vi "PDash New Event.vi"(8 "error in":errorcluster, 10 "Current Selection":T4, 11 "Project":refnum<class "Project.lvclass">) -> (0 "error out":errorcluster)   [LabVIEW 2020]
doc: "Panther Dashboard DQMH UI Template"
uses:
  Panther Dashboard.lvlib
  Class/Library/Library.lvclass
  Class/Project/Project.lvclass
  <vilib>/Delacor/Delacor QMH/Libraries/_Scripting Support/Request Scoping--enum.ctl
  <vilib>/Delacor/Delacor QMH/Libraries/_Scripting Support/dqmh_lib_DQMH Scripting Support.lvlib
  <vilib>/Delacor/Delacor QMH/Libraries/_Scripting Support/Module Type--enum.ctl
  Controls/Cancel.ctl
  Controls/Continue.ctl
  Class/VI/VI.lvclass
  <vilib>/Delacor/Delacor QMH/Libraries/_Scripting Support/Module Info--cluster.ctl
panel:
  out "error out 2":errorcluster
  in  "Module Info":T1
  in  "Event Info":T3
  in  "error in 2":errorcluster
  in  "Pre Set Dummy Arg":bool
  in  "Progress Title (\"New DQMH Event\")":string
  in  "Skip Post-Scripting Action (F)":bool
  out "Selected Module":string caption="Current Module Selection:"
  in  "Module Description":string caption="New Module Description"
  in  "New Module Path":path
  in  "Module Name":string caption="New Module Name"
  in  "Continue":T5
  in  "Cancel":T6
  # "Note: To Select the DQMH Default UIs, click the Gear Icon on the Panther Dashboard\nMain UI, and Uncheck the 'Use Panther Dashboard UIs' checkbox."
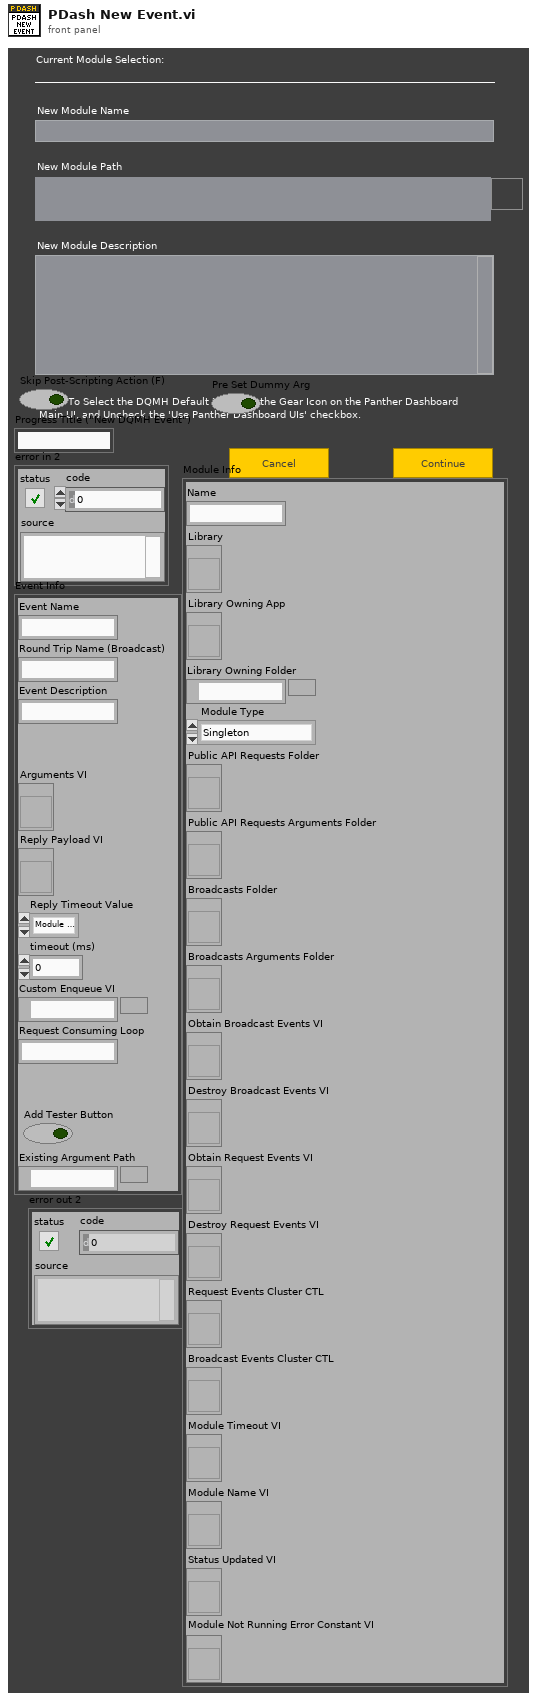
[diagram p1: front panel]
types:
  T1 = typedef "dqmh_lib_DQMH Scripting Support.lvlib/Module Info--cluster.ctl" = cluster{"Name":string, "Library":refnum<vi>, "Library Owning App":refnum<vi>, "Library Owning Folder":path, "Module Type":T2, "Public API Requests Folder":refnum<vi>, "Public API Requests Arguments Folder":refnum<vi>, "Broadcasts Folder":refnum<vi>, "Broadcasts Arguments Folder":refnum<vi>, "Obtain Broadcast Events VI":refnum<vi>, "Destroy Broadcast Events VI":refnum<vi>, "Obtain Request Events VI":refnum<vi>, "Destroy Request Events VI":refnum<vi>, "Request Events Cluster CTL":refnum<vi>, "Broadcast Events Cluster CTL":refnum<vi>, "Module Timeout VI":refnum<vi>, "Module Name VI":refnum<vi>, "Status Updated VI":refnum<vi>, "Module Not Running Error Constant VI":refnum<vi>}
  T2 = typedef "dqmh_lib_DQMH Scripting Support.lvlib/Module Type--enum.ctl" = enum16{"Singleton", "Cloneable"}
  T3 = typedef "dqmh_lib_DQMH Scripting Support.lvlib/Event Info (New)--cluster.ctl" = cluster{"Event Name":string, "Round Trip Name (Broadcast)":string, "Event Description":string, "Arguments VI":refnum<vi>, "Reply Payload VI":refnum<vi>, "Reply Timeout Value":enum32{"Module Timeout", "Custom"}, "timeout (ms)":i32, "Custom Enqueue VI":path, "Request Consuming Loop":string, "Add Tester Button":bool, "Existing Argument Path":path}
  T4 = cluster{"Library":refnum<class "Library.lvclass">, "VI":refnum<class "VI.lvclass">}
  T5 = typedef "Continue.ctl" = bool
  T6 = typedef "Cancel.ctl" = bool
  T7 = cluster{"Name":string, "Library":refnum<vi>, "Library Owning App":refnum<vi>, "Library Owning Folder":path, "Public API Requests Folder":refnum<vi>, "Public API Requests Arguments Folder":refnum<vi>, "Broadcasts Folder":refnum<vi>, "Broadcasts Arguments Folder":refnum<vi>, "Obtain Broadcast Events VI":refnum<vi>, "Destroy Broadcast Events VI":refnum<vi>, "Obtain Request Events VI":refnum<vi>, "Destroy Request Events VI":refnum<vi>, "Request Events Cluster CTL":refnum<vi>, "Broadcast Events Cluster CTL":refnum<vi>, "Module Timeout VI":refnum<vi>, "Module Name VI":refnum<vi>, "Status Updated VI":refnum<vi>, "Module Not Running Error Constant VI":refnum<vi>}
  T8 = cluster{"Event Name":string, "Round Trip Name (Broadcast)":string, "Event Description":string, "Arguments VI":refnum<vi>, "Reply Payload VI":refnum<vi>, "Reply Timeout Value":enum32{"Module Timeout", "Custom"}, "timeout (ms)":i32, "Custom Enqueue VI":path, "Request Consuming Loop":string, "Add Tester Button":bool, "Existing Argument Path":path}
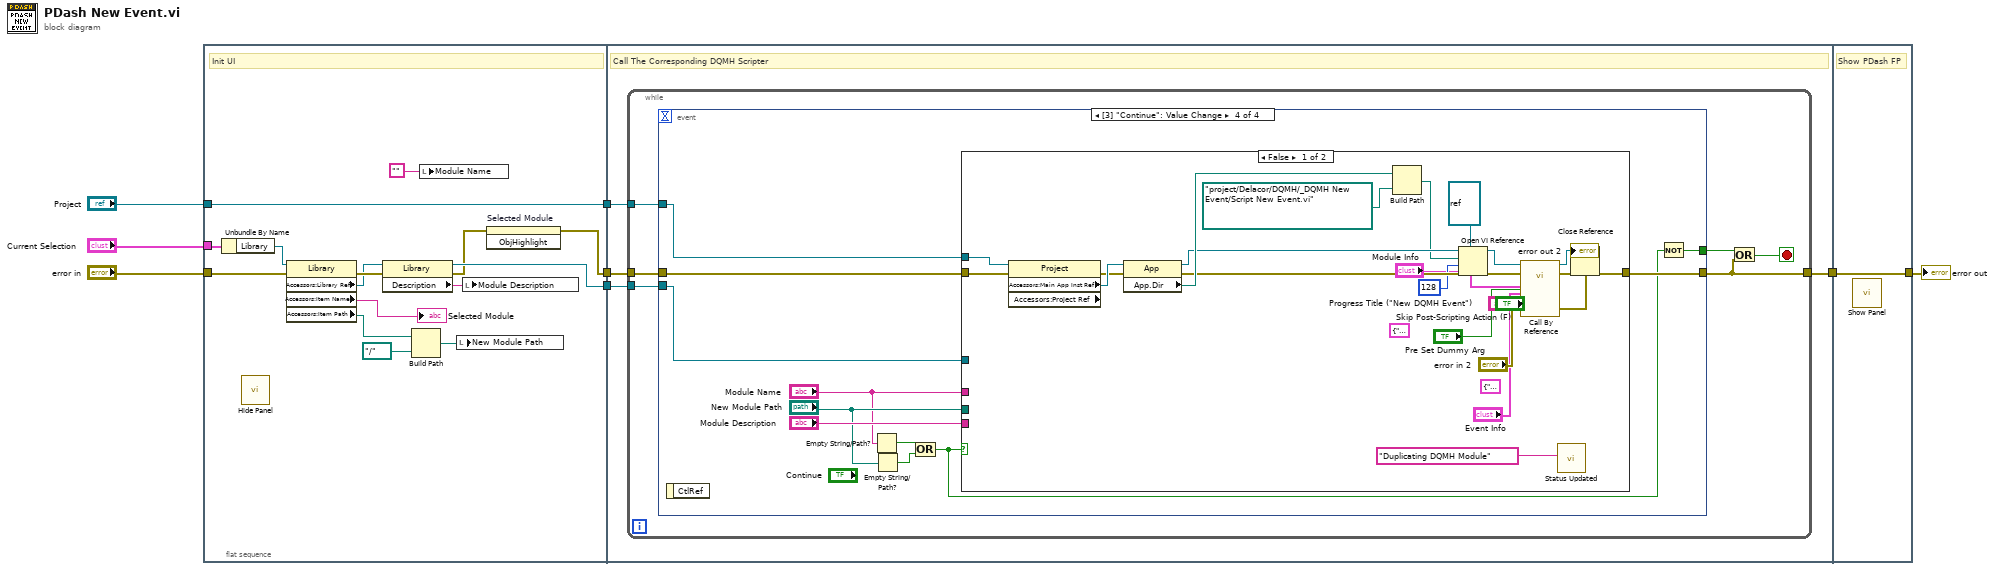
[diagram p0: block diagram]
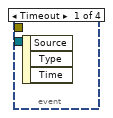
[diagram p2: hidden frame]
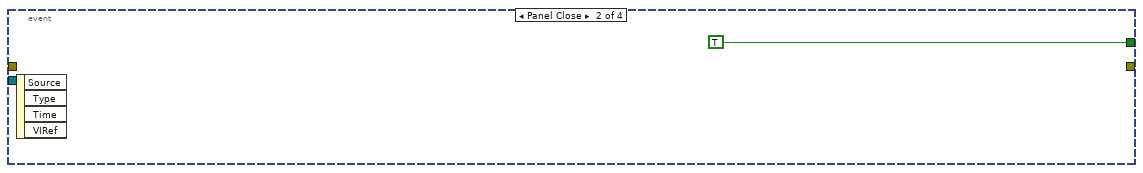
[diagram p3: hidden frame]
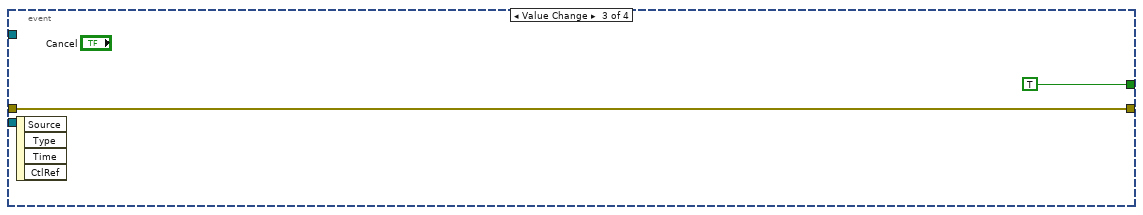
[diagram p4: hidden frame]
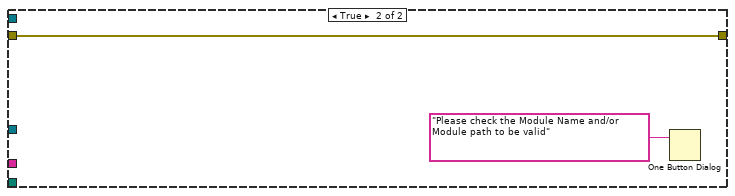
[diagram p5: hidden frame]
diagram:
  n1 = flat-sequence {
    tunnel: "Project" -> [w21]
    tunnel: [w21] -> w3
    tunnel: "error in" -> [w23]
    tunnel: [w9] -> w5
    tunnel: "Current Selection" -> [w20]
    tunnel: [w13] -> w1
    tunnel: [w27] -> w8
    tunnel: w3 -> [w25]
    tunnel: w5 -> [w26]
    tunnel: w1 -> [w24]
    tunnel: [w74] -> w7
    tunnel: w8 -> [w74]
    frame #0 {
      # "Init UI"
      n2 = Unbundle By Name(w20) -> ("Library"=w19:refnum<class "Library.lvclass">)
      n3 = call "Hide Panel.vi"() -> ()  [unwired: 11 in, 1 out]
      n4 = property class="Library"(reference=w19, error in=w23) -> (error out=w22:errorcluster, "Accessors:Library Ref"=w14:refnum<vi>, "Accessors:Item Name"=→"Selected Module":string, "Accessors:Item Path"=w16:path)  [unwired: 1 out]
      n5 = property class="Library"(reference=w14, error in=w22) -> (reference out=w13:refnum<vi>, error out=w10:errorcluster, "Description"=w12:string)
      n6 = Build Path(base path=w16, name or relative path=path "../..") -> (appended path=w18:path)
      n7 = local write "Module Name"("") -> ()
      n8 = local write "New Module Path"(w18) -> ()
      n9 = local write "Module Description"(w12) -> ()
      n10 = invoke on="Selected Module" class="Str" method="ObjHighlight"(error in=w10) -> (error out=w9:errorcluster)  [unwired: 2 in, 2 out]
    }
    frame #1 {
      # "Call The Corresponding DQMH Scripter"
      n11 = while {
        tunnel: [w28] -> w27
        tunnel: w25 -> [w31]
        tunnel: w26 -> [w33]
        tunnel: w24 -> [w30]
        stop <- w29 stop-if-true
        n12 = event shown="[3] \"Continue\": Value Change" {
          selector: _ -> [_ _ _ _]
          dyn-events: _ -> [_ _ _ _]
          timeout: _ -> [_ _ _ _]
          tunnel: [_ TRUE TRUE w45] -> w32
          tunnel: [_ _ w35 w38] -> w28
          tunnel: w31 -> [_ _ _ w41]
          tunnel: w33 -> [_ _ w35 w40]
          tunnel: w30 -> [_ _ _ w39]
          event Timeout {
            n13 = event-data() -> ()  [unwired: 1 in, 3 out]
          }
          event Panel Close {
            n14 = event-data() -> ()  [unwired: 1 in, 4 out]
          }
          event Value Change {
            n15 = event-data() -> ()  [unwired: 1 in, 4 out]
          }
          event Value Change {
            n16 = event-data() -> ()  [unwired: 1 in, 1 out]
            n17 = Empty String/Path?(string/path="Module Name") -> (empty?=w47:bool)
            n18 = Empty String/Path?(string/path="New Module Path") -> (empty?=w46:bool)
            n19 = Or(x=w47, y=w46) -> (x .or. y?=w37:bool)
            n20 = case shown="False" w37 {
              tunnel: "Module Description" -> [_ _]
              tunnel: "New Module Path" -> [_ _]
              tunnel: "Module Name" -> [_ _]
              tunnel: w41 -> [w60 _]
              tunnel: w40 -> [w59 w72]
              tunnel: w39 -> [_ _]
              tunnel: [w55 w72] -> w38
              frame False {
                (unwired) T7 {"Name"="", "Library"=refnum, "Library Owning App"=refnum, "Library Owning Folder"=path "", "Public API Requests Folder"=refnum, "Public API Requests Arguments Folder"=refnum, "Broadcasts Folder"=refnum, "Broadcasts Arguments Folder"=refnum, "Obtain Broadcast Events VI"=refnum, "Destroy Broadcast Events VI"=refnum, "Obtain Request Events VI"=refnum, "Destroy Request Events VI"=refnum, "Request Events Cluster CTL"=refnum, "Broadcast Events Cluster CTL"=refnum, "Module Timeout VI"=refnum, "Module Name VI"=refnum, "Status Updated VI"=refnum, "Module Not Running Error Constant VI"=refnum} ("Module Info")
                (unwired) T8 {"Event Name"="", "Round Trip Name (Broadcast)"="", "Event Description"="", "Arguments VI"=refnum, "Reply Payload VI"=refnum, "Reply Timeout Value"=enum."Module Timeout", "timeout (ms)"=0, "Custom Enqueue VI"=path "", "Request Consuming Loop"="", "Add Tester Button"=FALSE, "Existing Argument Path"=path ""} ("Event Info")
                n21 = property class="Project" props=["Accessors:Main App Inst Ref", "Accessors:Project Ref"](reference=w60, error in=w59) -> (error out=w64:errorcluster, "Accessors:Main App Inst Ref"=w69:refnum<vi>)  [unwired: 2 out]
                n22 = property class="App"(reference=w69, error in=w64) -> (reference out=w67:refnum<vi>, error out=w63:errorcluster, "App.Dir"=w68:path)
                n23 = Build Path(base path=w68, name or relative path=path "project/Delacor/DQMH/_DQMH New Event/Script New Event.vi") -> (appended path=w65:path)
                n24 = Open VI Reference(type specifier VI Refnum (for type only)=refnum<vi> refnum, application reference (local)=w67, vi path=w65, options=128, error in (no error)=w63) -> (vi reference=w70:refnum<vi>, error out=w61:errorcluster)  [unwired: 1 in]
                n25 = call-by-ref "?"(reference=w70, error in=w61, "Skip Post-Scripting Action (F)"="Skip Post-Scripting Action (F)", "Progress Title (\"New DQMH Event\")"="Progress Title (\"New DQMH Event\")", "Pre Set Dummy Arg"="Pre Set Dummy Arg", "error in"="error in 2", "Event Info"="Event Info", "Module Info"="Module Info") -> (reference out=w66:refnum<vi>, error out=w62:errorcluster, 0:"error out"=→"error out 2":errorcluster)  [unwired: 5 in]
                n26 = call "Status Updated.vi"("Status"="Duplicating DQMH Module") -> ()  [unwired: 10 in, 1 out]
                n27 = Close Reference(reference=w66, error in (no error)=w62) -> (error out=w55:errorcluster)
              }
              frame True {
                n28 = One Button Dialog(message="Please check the Module Name and/or Module path to be valid") -> ()  [unwired: 1 in, 1 out]
              }
            }
            n29 = Not(x=w37) -> (.not. x?=w45:bool)
          }
        }
        n30 = Or(x=w32, y=w28) -> (x .or. y?=w29:bool)
      }
    }
    frame #2 {
      # "Show PDash FP"
      n31 = call "Show Panel.vi"() -> ()  [unwired: 11 in, 1 out]
    }
  }
  "error out" <- w7
